vi "is_zero.vi"(8 "error in (no error)":errorcluster, 11 "SpaceVector in":refnum<class "SpaceVector.lvclass">) -> (0 "error out":errorcluster, 2 "zero?":bool, 3 "SpaceVector out":refnum<class "SpaceVector.lvclass">)   [LabVIEW 2010, in "SpaceVector.lvclass"]
uses:
  SpaceVector.lvclass
  SpaceVector.lvclass/SpaceVector.ctl
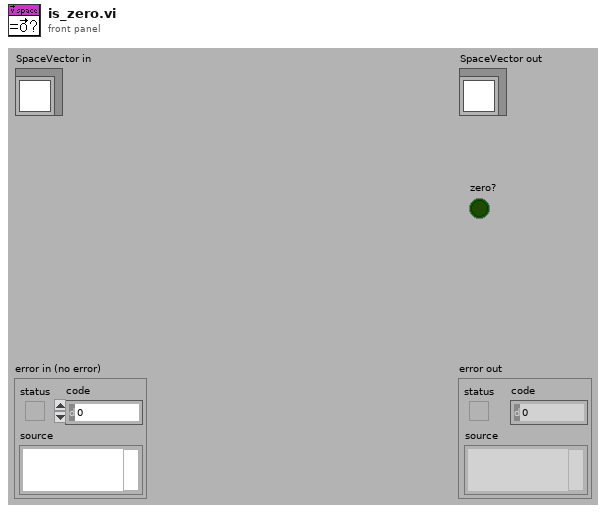
[diagram p1: front panel]
types:
  T1 = typedef "space_vector_array.ctl" = dbl[unit][]
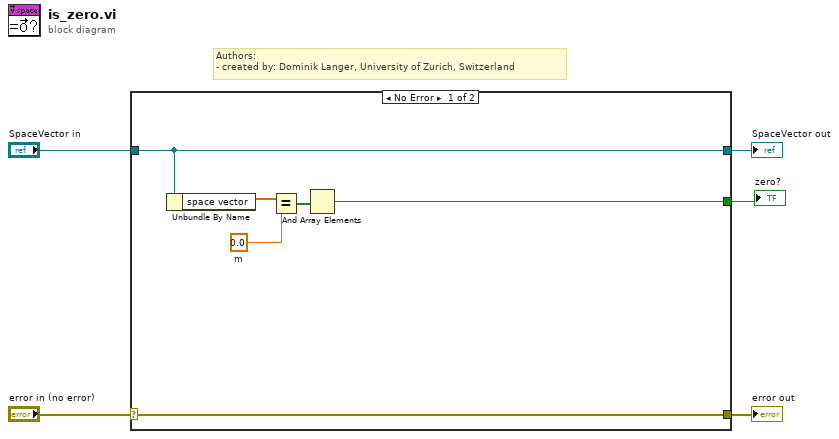
[diagram p0: block diagram]
diagram:
  # "Authors: \n- created by: Dominik Langer, University of Zurich, Switzerland"
  n1 = case shown="No Error" "error in (no error)" {
    selector: "error in (no error)" -> [w11 w13]
    tunnel: [w11 w13] -> w4
    tunnel: [w10 w12] -> w2
    tunnel: "SpaceVector in" -> [w10 w12]
    tunnel: [w6 _] -> w1
    frame No Error {
      w8 = dbl[unit] 0.0  # m
      n2 = Unbundle By Name(w10) -> ("space vector"=w9:T1)
      n3 = Equal?(x=w9, y=w8) -> (x = y?=w7:bool[])
      n4 = And Array Elements(Boolean array=w7) -> (logical AND=w6:bool)
    }
    frame Error {
    }
  }
  "error out" <- w4
  "SpaceVector out" <- w2
  "zero?" <- w1
